vi "Minimize Memory Example.vi"() -> ()   [LabVIEW 2020]
doc: "An example which demonstrates how to minimize memory use when reading large audio files into memory."
uses:
  071ebbf0-815d-4e33-b582-2127f939b57d.vi
  39075c41-dad1-4b1e-9ff0-30057265b9d9.vi
  Private/Get Basic Audio File Info.vi
  Private/Result To Error.vi
  071ebbf0-815d-4e33-b582-2127f939b57d.vi/779dfdfd-1b42-4cf4-8001-66d3dd167625.vi
  071ebbf0-815d-4e33-b582-2127f939b57d.vi/55d550d4-9624-414e-aebd-6e02b5081896.vi
  Private/Audio File Refnum To Value.vi
  39075c41-dad1-4b1e-9ff0-30057265b9d9.vi/779dfdfd-1b42-4cf4-8001-66d3dd167625.vi
  39075c41-dad1-4b1e-9ff0-30057265b9d9.vi/55d550d4-9624-414e-aebd-6e02b5081896.vi
  071ebbf0-815d-4e33-b582-2127f939b57d.vi/55d550d4-9624-414e-aebd-6e02b5081896.vi/4b7b629c-2e91-4160-9820-a26af8f6e677.vi
  39075c41-dad1-4b1e-9ff0-30057265b9d9.vi/55d550d4-9624-414e-aebd-6e02b5081896.vi/4b7b629c-2e91-4160-9820-a26af8f6e677.vi
  Audio Files/Polymorphic VIs/Get Audio File Info (Path).vi
  Audio Files/Polymorphic VIs/Open Audio File Read (Path).vi
  <vilib>/Utility/Data Type/Get Numeric Information.vi
  <vilib>/Utility/error.llb/Error Cluster From Error Code.vi
  G-Audio.lvlib
panel:
  in  "Minimize Memory":bool
  out "Memory Allocated":string
  out "error out":errorcluster
  # "Instructions:\n1. Run the VI.\n2. Select a large audio file to read.\n3. Observe the Memory Allocated.\n4. Toggle the Minimize Memory flag,\n    and run the VI again.\n5. Select the same audio file and observe the\n    Memory Allocated."
  # "When the audio data format is a 2D array, additional memory will be allocated when converting the interleaved 1D array to a 2D array. This example shows one method of minimizing the memory footprint. It also applies to data type conversion (e.g. source is I16, and format requested is DBL).\n\nWhen using the file reading method where Minimize Memory is unchecked, LabVIEW will eventually release or reuse the extra allocated memory. This method is safe to use for smaller files, but larger files may run into out of memory errors, especially under LabVIEW 32-bit.\n\nIf the audio data format is a 1D waveform array, no additional memory allocations are incurred as LabVIEW reuses the space already allocated to the original 1D array. Additional memory will still be allocated if the native audio file data type (e.g. I16) differs from the requested audio data type.\n\nOther tips for reducing memory use:\n* Read audio files in their native data type.\n* Avoid using 64-bit DBL types when reading data, as most audio data is only 16-bit or 24-bit. Only convert to DBL when processing audio data.\n* Avoid loading the entire file into memory if possible. Instead read and process it in blocks from disk."
  # "G"
  # "-Audio"
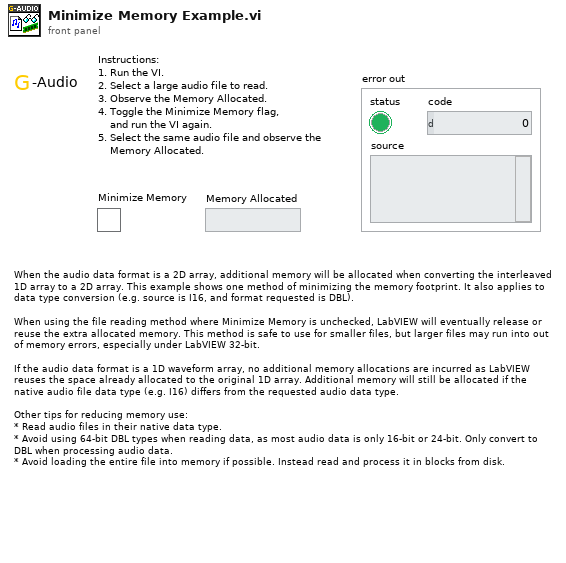
[diagram p1: front panel]
types:
  T1 = typedef "G-Audio.lvlib/Audio File Info.ctl" = cluster{"Sample Rate (Hz)":u32, "Channels":u32, "Bit Depth":u32}
  T2 = typedef "G-Audio.lvlib/Audio File Refnum.ctl" = refnum<file>
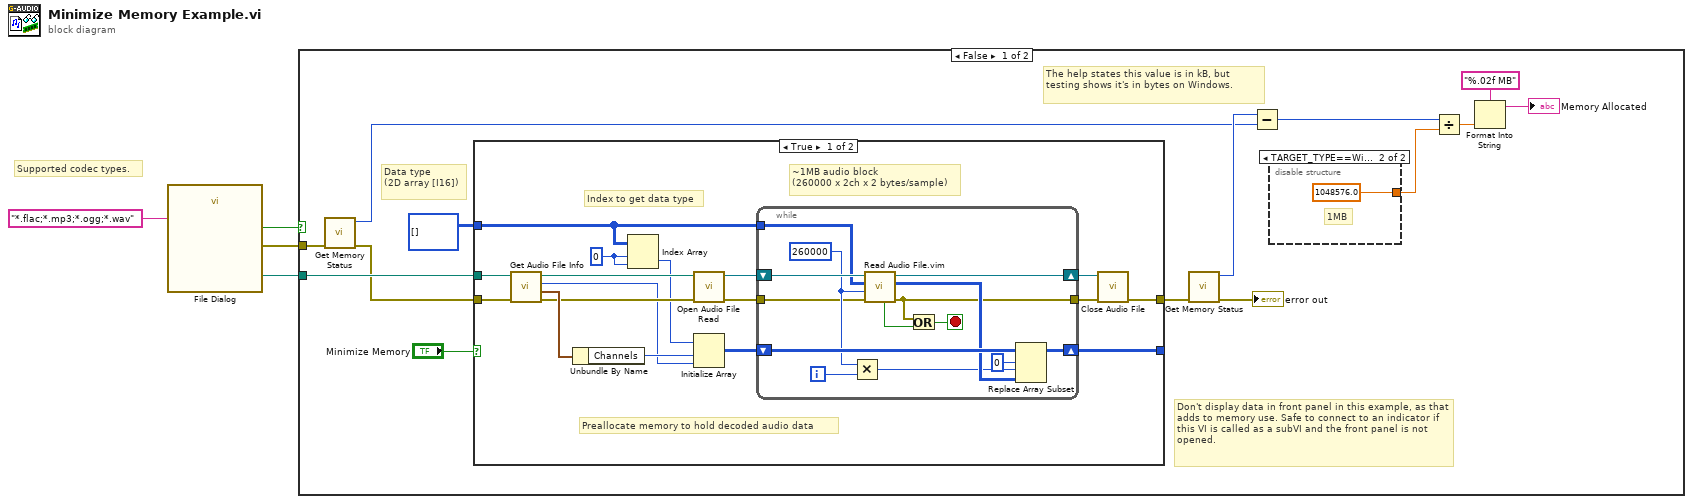
[diagram p0: block diagram]
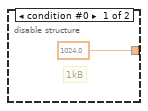
[diagram p2: hidden frame]
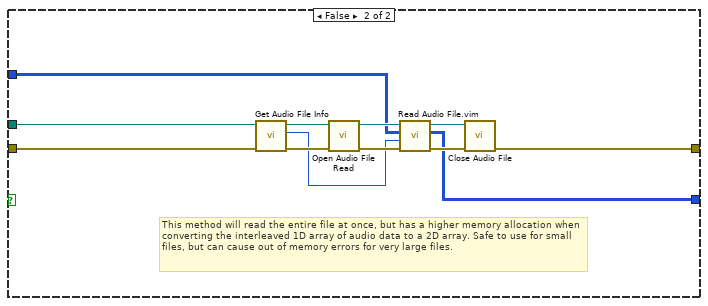
[diagram p3: hidden frame]
diagram:
  # "Supported codec types."
  n1 = call "File Dialog"("pattern (all files)"="*.flac;*.mp3;*.ogg;*.wav") -> ("selected path"=w3:path, "cancelled"=w1:bool, "error out"=w2:errorcluster)  [unwired: 11 in, 1 out]
  n2 = case shown="False" w1 {
    tunnel: w3 -> [w18 _]
    tunnel: w2 -> [w16 _]
    frame False {
      # "The help states this value is in kB, but testing shows it's in bytes on Windows."
      # "Data type\n(2D array [I16])"
      # "Don't display data in front panel in this example, as that adds to memory use. Safe to connect to an indicator if this VI is called as a subVI and the front panel is not opened."
      n3 = call <vilib>:"Get Memory Status.vi"("error in (no error)"=w16) -> ("error out"=w17:errorcluster, "memory allocated for LabVIEW"=w6:u64)  [unwired: 7 in, 2 out]
      n4 = case shown="True" "Minimize Memory" {
        tunnel: w18 -> [w37 w63]
        tunnel: w17 -> [w26 w56]
        tunnel: [w25 w55] -> w15
        tunnel: [w24 w53] -> _
        tunnel: i16[][] [] ("initialized array") -> [w23 w52]
        frame True {
          w22 = 0 ("index (row)")
          # "Index to get data type"
          # "Preallocate memory to hold decoded audio data"
          # "~1MB audio block\n(260000 x 2ch x 2 bytes/sample)"
          n5 = call-poly "Get Audio File Info.vi"("error in (no error)"=w26, "Path In"=w37) -> ("error out"=w33:errorcluster, "Audio File Info"=w36:T1, "PCM Frame Length"=w30:u64, "Path Out"=w34:path)  [unwired: 5 in, 1 out]
          n6 = Unbundle By Name(w36) -> ("Channels"=w35:u32)
          n7 = Index Array(array=w23, index (row)=w22, index (col)=w22) -> (element=w21:i16)
          n8 = call-poly "Open Audio File Read.vi"("error in (no error)"=w33, "Path"=w34) -> ("error out"=w27:errorcluster, "Audio File Refnum"=w32:T2)  [unwired: 8 in]
          n9 = Initialize Array(w21, w35, w30) -> (w31:i16[][])
          n10 = while {
            shift-right: [w43] -> w24
            shift-left: w31 -> [w49]
            shift-right: [w42] -> w29
            shift-left: w32 -> [w51]
            tunnel: w23 -> [w50]
            tunnel: [w38] -> w28
            tunnel: w27 -> [w41]
            i -> [w46]
            stop <- w39 stop-if-true
            w45 = u64 260000 ("Frames To Read")
            n11 = Multiply(x=w45, y=w46) -> (x*y=w44:u64)
            n12 = call "Read Audio File.vim"("error in (no error)"=w41, "Frames To Read"=w45, "Data Format"=w50, "Audio File Refnum In"=w51) -> ("error out"=w38:errorcluster, "Audio Data"=w48:i16[][], "Audio File Refnum Out"=w42:T2, "End of File?"=w40:bool)  [unwired: 3 in, 1 out]
            n13 = Or(x=w38, y=w40) -> (x .or. y?=w39:bool)
            n14 = Replace Array Subset(array=w49, new element=w48, index (row)=0 ("disabled index (row)"), index (col)=w44) -> (w43:i16[][])
          }
          n15 = call "Close Audio File.vi"("error in (no error)"=w28, "Audio File Refnum In"=w29) -> ("error out"=w25:errorcluster)  [unwired: 9 in]
        }
        frame False {
          # "This method will read the entire file at once, but has a higher memory allocation when converting the interleaved 1D array of audio data to a 2D array. Safe to use for small files, but can cause out of memory errors for very large files."
          n16 = call-poly "Get Audio File Info.vi"("error in (no error)"=w56, "Path In"=w63) -> ("error out"=w61:errorcluster, "PCM Frame Length"=w54:u64, "Path Out"=w62:path)  [unwired: 5 in, 2 out]
          n17 = call-poly "Open Audio File Read.vi"("error in (no error)"=w61, "Path"=w62) -> ("error out"=w57:errorcluster, "Audio File Refnum"=w60:T2)  [unwired: 8 in]
          n18 = call "Read Audio File.vim"("error in (no error)"=w57, "Frames To Read"=w54, "Data Format"=w52, "Audio File Refnum In"=w60) -> ("error out"=w58:errorcluster, "Audio Data"=w53:i16[][], "Audio File Refnum Out"=w59:T2)  [unwired: 3 in, 2 out]
          n19 = call "Close Audio File.vi"("error in (no error)"=w58, "Audio File Refnum In"=w59) -> ("error out"=w55:errorcluster)  [unwired: 9 in]
        }
      }
      n20 = call <vilib>:"Get Memory Status.vi"("error in (no error)"=w15) -> ("error out"=→"error out":errorcluster, "memory allocated for LabVIEW"=w13:u64)  [unwired: 7 in, 2 out]
      n21 = Subtract(x=w13, y=w6) -> (x-y=w12:u64)
      n22 = disable-structure shown="TARGET_TYPE==Windows" {
        disable-tunnel: [1024.0 ("y") 1048576.0 ("y")] -> w11
        frame condition #0 {
          # "1kB"
        }
        frame condition #1 (active) {
          # "1MB"
        }
      }
      n23 = Divide(x=w12, y=w11) -> (x/y=w10:dbl)
      n24 = Format Into String(format string="%.02f MB", w10) -> (resulting string=→"Memory Allocated":string)  [unwired: 2 in, 1 out]
    }
    frame True {
    }
  }
